vi "RSZVB Set Trace Scale Divisions.vi"(7 "Scale Divisions (10.0)":dbl=10.0 format="%^.3e", 8 "error in (no error)":errorcluster {"code" format="%.0x"}, 9 "Window (Trace) (1)":i32=1, 10 "Window (1)":i32=1, 11 "VISA session":refnum<visa-resource-name>) -> (0 "error out":errorcluster {"code" format="%.0x"}, 3 "dup VISA session":refnum<visa-resource-name>)   [LabVIEW 2011]
doc: "This VI sets the value of the vertical diagram divisions in Cartesian diagrams.\n\nScale /Div corresponds to the increment between two consecutive grid lines. The unit depends on the display format: dB for display format dB Mag, degrees for Phase and Unwrapped Phase, ns for Delay, U (units) for all other (dimensionless) formats.\n\nNote(s):\n\n(1) Window:\nNumber of an existing diagram area (defined by means of DISPlay:WINDow<Wnd>:STATe ON). \n \n(2) Window (Trace):\nExisting trace number, assigned by means of DISPlay:WINDow<Wnd>:TRACe<WndTr>:FEED.\n\nRemote-control command(s):\nDISPlay:WINDow<Wnd>:TRACe<WndTr>:Y[:SCALe]:PDIVision <numeric_value>"
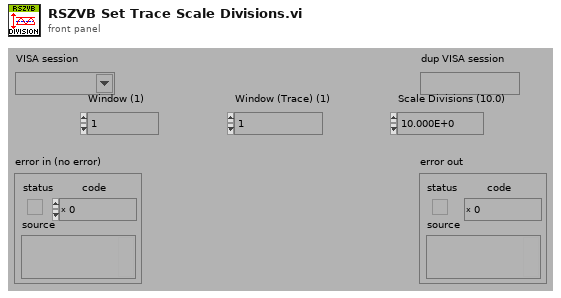
[diagram p1: front panel]
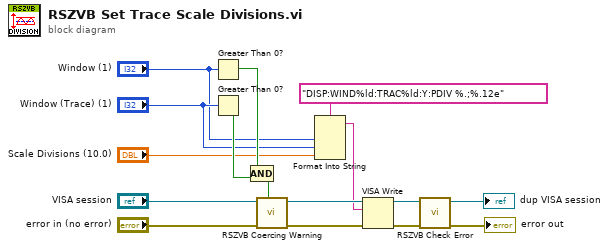
[diagram p0: block diagram]
diagram:
  n1 = Greater Than 0?(x="Window (1)") -> (x > 0?=w4:bool)
  n2 = Greater Than 0?(x="Window (Trace) (1)") -> (x > 0?=w5:bool)
  n3 = Compound Arithmetic op=AND(w4, w5) -> (w11:bool)
  n4 = call "RSZVB Coercing Warning.vi"("In Range?"=w11, "error in (no error)"="error in (no error)", "VISA session"="VISA session") -> ("error out"=w14:errorcluster, "dup VISA session"=w15:refnum<visa-resource-name>)  [unwired: 7 in]
  n5 = Format Into String(format string="DISP:WIND%ld:TRAC%ld:Y:PDIV %.;%.12e", "Window (1)", "Window (Trace) (1)", "Scale Divisions (10.0)") -> (resulting string=w10:string)  [unwired: 2 in, 1 out]
  n6 = VISA Write(VISA resource name=w15, write buffer=w10, error in (no error)=w14) -> (VISA resource name out=w12:refnum<visa-resource-name>, error out=w13:errorcluster)  [unwired: 1 out]
  n7 = call "RSZVB Check Error.vi"("error in (no error)"=w13, "VISA session"=w12) -> ("error out"=→"error out":errorcluster, "dup VISA session"=→"dup VISA session":refnum<visa-resource-name>)  [unwired: 8 in]
